vi "Differential Pressure Release Valve Test DAA.vi"(8 "error in (no error)":errorcluster, 10 "Model in":refnum<class "Model.lvclass">, 11 "Test Actuator State in":refnum<class "Test Actuator State.lvclass">) -> (0 "error out":errorcluster, 1 "Pass":bool, 2 "Model out":refnum<class "Model.lvclass">, 3 "Test Actuator State out":refnum<class "Test Actuator State.lvclass">)   [LabVIEW 2016]
uses:
  Model/Model/Model.lvclass
  Typedefs/ActuatorSetPoints.ctl
  <vilib>/platform/TimedLoop/XDataNode/XDataNode.xnode
  <vilib>/Platform/TimedLoop/XDataNode/nitl_modes.ctl
  <vilib>/Platform/TimedLoop/XDataNode/XDNodeRunTimeDep.lvlib
  <vilib>/Platform/TimedLoop/XDataNode/wakeup.ctl
  <vilib>/Platform/TimedLoop/XDataNode/timing_clust.ctl
  Test Actuator State.lvclass
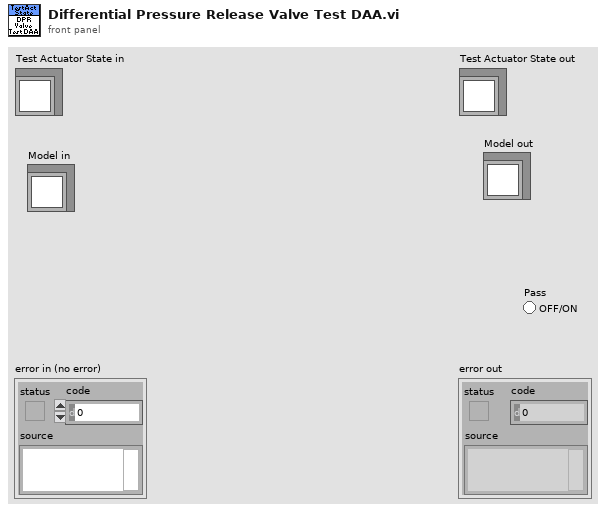
[diagram p1: front panel]
types:
  T1 = typedef "DifferentialPressureReleaseValveTestSettings.ctl" = cluster{"Max Over Force (N)":dbl, "Max Moment (NM)":dbl, "Process Time (s)":dbl, "Sample Time (s)":dbl}
  T2 = typedef "ForcePair.ctl" = cluster{"Axial Force":dbl, "Lateral Force":dbl}
  T3 = typedef "FullForceScanSettings.ctl" = cluster{"Force Tolerance (N)":dbl, "DAA Force Set Points":T2[], "Process Time (s)":dbl, "Sample Time (s)":dbl, "Max Moment (NM)":dbl, "SAA Force Set Points":T2[]}
  T4 = cluster{"Top Left":T2, "Top Right":T2, "Bottom Right":T2, "Bottom Left":T2}
  T5 = typedef "ActuatorSetPoints.ctl" = cluster{"Axial Force":dbl, "Lateral Force":dbl, "FC1 Force":dbl, "FC2 Force":dbl}
  T6 = typedef "XDNodeRunTimeDep.lvlib/timing_clust.ctl" = cluster{"Expected End [f-1]":u64, "Actual End [f-1]":u64, "Finished Late? [f-1]":bool, "Expected End [i-1]":u64, "Actual End [i-1]":u64, "Finished Late? [i-1]":bool, "Expected Start [i]":u64, "Actual Start [i]":u64, "Expected Start [f]":u64, "Actual Start [f]":u64, "Source Name":string, "Structure Name":string, "Period":i64, "Deadline":i64, "Offset":i64, "Start":i64, "Priority":i32, "Timeout":i32, "Mode":T7, "Wakeup Reason":T8, "Error":errorcluster, "Source Type":string, "Secondary Source Type":string, "Global End Time":u64, "Global Start Time":u64, "Frame Duration":u64, "Iteration Duration":u64, "Assigned CPU":i32, "I/O Scan Engine Mode":u32}
  T7 = typedef "XDNodeRunTimeDep.lvlib/nitl_modes.ctl" = enum32{"No Change", "Process missed periods, maintain original phase", "Discard missed periods, maintain original phase", "Process missed periods, ignore original phase", "Discard missed periods, ignore original phase"}
  T8 = typedef "XDNodeRunTimeDep.lvlib/wakeup.ctl" = enum32{"Normal", "Aborted", "Asynchronous wakeup", "Timing source error", "Timed loop error", "Timeout"}
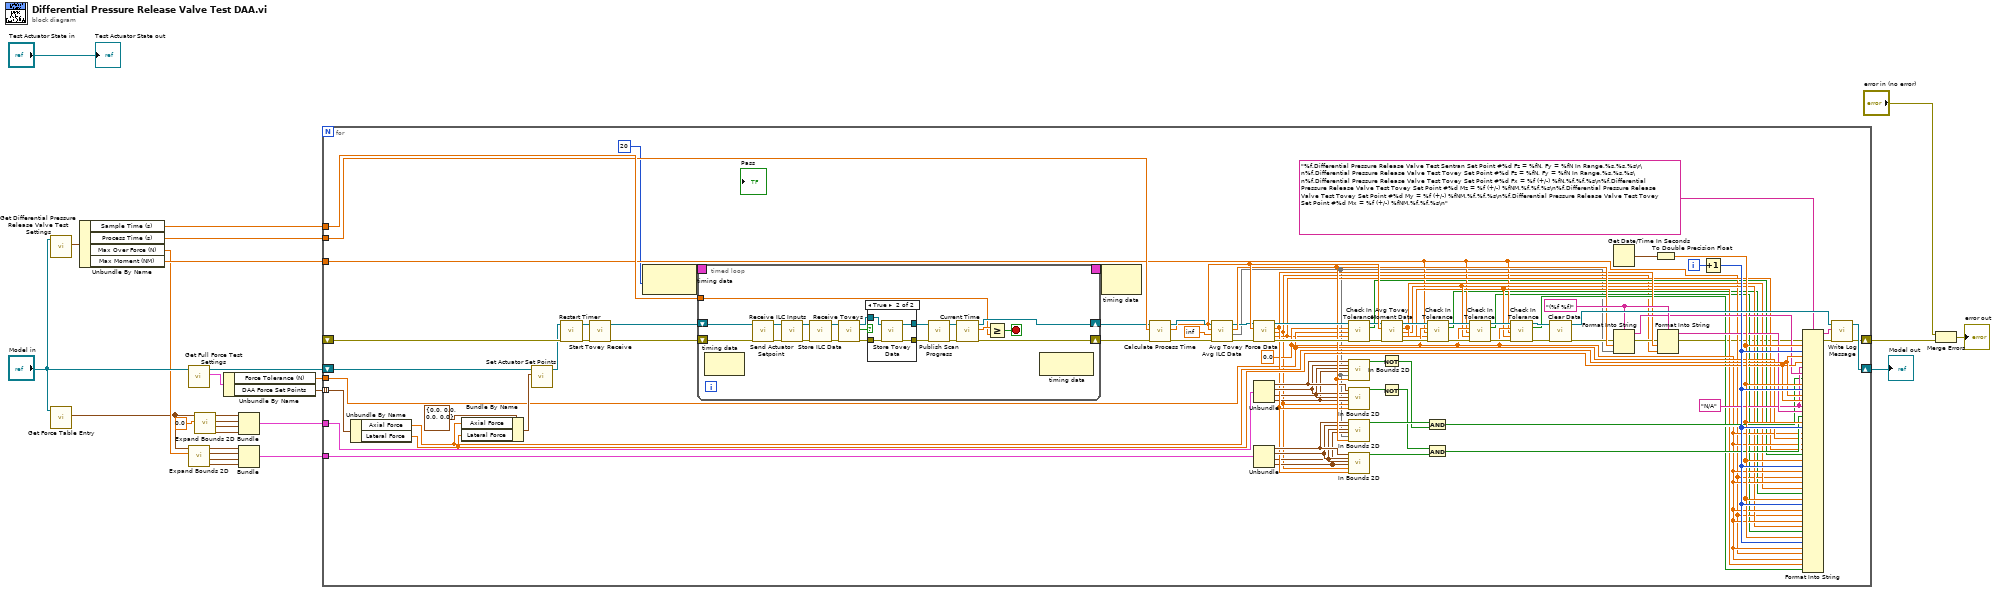
[diagram p0: block diagram]
diagram:
  n1 = call-dynamic "Get Differential Pressure Release Valve Test Settings.vi"("Model in"="Model in") -> ("Differential Pressure Release Valve Test Settings"=w16:T1)  [unwired: 9 in, 1 out]
  n2 = call "Get Force Table Entry.vi"("Model in"="Model in") -> ("Entry"=w8:T2[])  [unwired: 8 in, 2 out]
  n3 = Unbundle By Name(w16) -> ("Sample Time (s)"=w25:dbl, "Process Time (s)"=w24:dbl, "Max Over Force (N)"=w15:dbl, "Max Moment (NM)"=w19:dbl)
  n4 = call "Get Full Force Test Settings.vi"("Model in"="Model in") -> ("Full Force Test Settings"=w18:T3, "Model out"=w26:refnum<class "Model.lvclass">)  [unwired: 9 in]
  n5 = call "Expand Bounds 2D.vi"("Tolerance (N)"=w15, "Entry"=w8) -> ("Bottom Left"=w10:T2, "Bottom Right"=w11:T2, "Top Right"=w12:T2, "Top Left"=w13:T2)  [unwired: 6 in]
  n6 = call "Expand Bounds 2D.vi"("Tolerance (N)"=0.0, "Entry"=w8) -> ("Bottom Left"=w3:T2, "Bottom Right"=w4:T2, "Top Right"=w5:T2, "Top Left"=w6:T2)  [unwired: 6 in]
  n7 = Unbundle By Name(w18) -> ("Force Tolerance (N)"=w1:dbl, "DAA Force Set Points"=w14:T2[])
  n8 = Bundle("Top Left"=w6, "Top Right"=w5, "Bottom Right"=w4, "Bottom Left"=w3) -> (w2:T4)  [unwired: 1 in]
  n9 = Bundle("Top Left"=w13, "Top Right"=w12, "Bottom Right"=w11, "Bottom Left"=w10) -> (w9:T4)  [unwired: 1 in]
  n10 = for {
    tunnel: w14 -> [w99] mode=indexing
    shift-right: [w109] -> w21
    shift-left: w26 -> [w113]
    tunnel: w25 -> [w112]
    tunnel: w24 -> [w95]
    shift-right: [w96] -> w20
    shift-left: _ -> [w111]
    tunnel: w19 -> [w45]
    tunnel: w9 -> [w74]
    tunnel: w2 -> [w73]
    tunnel: w1 -> [w52]
    i -> [w106]
    w63 = "N/A" ("input 5")
    w67 = "(%f %f)" ("format string")
    w50 = 0.0
    n11 = Unbundle By Name(w99) -> ("Axial Force"=w69:dbl, "Lateral Force"=w68:dbl)
    n12 = Bundle By Name(cluster=T5 {"Axial Force"=0.0, "Lateral Force"=0.0, "FC1 Force"=0.0, "FC2 Force"=0.0} ("Actuator Set Points"), "Axial Force"=w69, "Lateral Force"=w68) -> (w100:T5)
    n13 = call "Set Actuator Set Points.vi"("Actuator Set Points"=w100, "Model in"=w113) -> ("Model out"=w101:refnum<class "Model.lvclass">)  [unwired: 9 in]
    n14 = call "Restart Timer.vi"("error in (no error)"=w111, "Model in"=w101) -> ("error out"=w104:errorcluster, "Model out"=w105:refnum<class "Model.lvclass">)  [unwired: 8 in]
    n15 = call "Start Tovey Receive.vi"("error in (no error)"=w104, "Model in"=w105) -> ("error out"=w102:errorcluster, "Model out"=w103:refnum<class "Model.lvclass">)  [unwired: 8 in]
    n16 = node-c288(i64 20 ("Period")) -> (w30:T6)
    n17 = timed-loop {
      shift-right: [w128] -> w94
      shift-left: w103 -> [w134]
      shift-right: [w127] -> w92
      shift-left: w102 -> [w131]
      tunnel: w112 -> [w125]
      timing: w30 -> [_]
      timing-out: [_] -> w29
      stop <- w124 stop-if-true
      n18 = node-c288() -> ()  [unwired: 1 in, 1 out]
      n19 = call "Send Actuator Setpoint.vi"("error in (no error)"=w131, "Model in"=w134) -> ("error out"=w130:errorcluster, "Model out"=w133:refnum<class "Model.lvclass">)  [unwired: 8 in]
      n20 = call "Receive ILC Inputs.vi"("error in (no error)"=w130, "Model in"=w133) -> ("error out"=w129:errorcluster, "Model out"=w132:refnum<class "Model.lvclass">)  [unwired: 8 in]
      n21 = call "Store ILC Data.vi"("error in (no error)"=w129, "Model in"=w132) -> ("error out"=w122:errorcluster, "Model out"=w123:refnum<class "Model.lvclass">)  [unwired: 8 in]
      n22 = call "Receive Toveys.vi"("error in (no error)"=w122, "Model in"=w123) -> ("error out"=w120:errorcluster, "Data Received"=w119:bool, "Model out"=w121:refnum<class "Model.lvclass">)  [unwired: 7 in]
      n23 = case shown="True" w119 {
        tunnel: w121 -> [w138 w142]
        tunnel: w120 -> [w137 w141]
        tunnel: [w137 w140] -> w115
        tunnel: [w138 w139] -> w118
        frame False {
        }
        frame True {
          n24 = call "Store Tovey Data.vi"("error in (no error)"=w141, "Model in"=w142) -> ("error out"=w140:errorcluster, "Model out"=w139:refnum<class "Model.lvclass">)  [unwired: 8 in]
        }
      }
      n25 = call "Publish Scan Progress.vi"("error in (no error)"=w115, "Model in"=w118) -> ("error out"=w116:errorcluster, "Model out"=w117:refnum<class "Model.lvclass">)  [unwired: 8 in]
      n26 = call "Current Time.vi"("error in (no error)"=w116, "Model in"=w117) -> ("error out"=w127:errorcluster, "Time"=w126:dbl, "Model out"=w128:refnum<class "Model.lvclass">)  [unwired: 7 in]
      n27 = Greater Or Equal?(x=w126, y=w125) -> (x >= y?=w124:bool)
      n28 = node-c288() -> ()  [unwired: 1 in, 1 out]
    }
    n29 = node-c288(w29) -> ()  [unwired: 1 out]
    n30 = call "Calculate Process Time.vi"("error in (no error)"=w92, "Seconds"=w95, "Model in"=w94) -> ("error out"=w91:errorcluster, "Time"=w90:dbl, "Model out"=w93:refnum<class "Model.lvclass">)  [unwired: 6 in]
    n31 = call "Avg ILC Data.vi"("error in (no error)"=w91, "Before This Time"=inf, "After This Time"=w90, "Model in"=w93) -> ("error out"=w89:errorcluster, 1:w32, "Force"=w66:dbl, "Model out"=w51:refnum<class "Model.lvclass">)  [unwired: 4 in]
    n32 = call "Avg Tovey Force Data.vi"("Model in"=w51, "After This Time"=w90, "error in (no error)"=w89) -> ("Model out"=w86:refnum<class "Model.lvclass">, "Fz"=w57:dbl, "Fy"=w33:dbl, "Fx"=w49:dbl, "error out"=w85:errorcluster)  [unwired: 8 in]
    n33 = Unbundle(w73) -> ("Top Left"=w59:T2, "Top Right"=w58:T2, "Bottom Right"=w35:T2, "Bottom Left"=w34:T2)
    n34 = Unbundle(w74) -> ("Top Left"=w61:T2, "Top Right"=w60:T2, "Bottom Right"=w37:T2, "Bottom Left"=w36:T2)
    n35 = call "Check In Tolerance.vi"("Model in"=w86, "Expected"=w50, "Tolerance"=w52, "Actual"=w49, "error in (no error)"=w85) -> ("Model out"=w83:refnum<class "Model.lvclass">, "Pass"=w41:bool, "error out"=w84:errorcluster)  [unwired: 8 in]
    n36 = call "In Bounds 2D.vi"("Top Left"=w59, "Top Right"=w58, "Bottom Right"=w35, "Bottom Left"=w34, "Lateral"=w32, "Axial"=w66) -> ("InBounds"=w72:bool)  [unwired: 13 in]
    n37 = call "In Bounds 2D.vi"("Top Left"=w59, "Top Right"=w58, "Bottom Right"=w35, "Bottom Left"=w34, "Lateral"=w33, "Axial"=w57) -> ("InBounds"=w56:bool)  [unwired: 13 in]
    n38 = call "In Bounds 2D.vi"("Top Left"=w61, "Top Right"=w60, "Bottom Right"=w37, "Bottom Left"=w36, "Lateral"=w32, "Axial"=w66) -> ("InBounds"=w71:bool)  [unwired: 13 in]
    n39 = call "In Bounds 2D.vi"("Top Left"=w61, "Top Right"=w60, "Bottom Right"=w37, "Bottom Left"=w36, "Lateral"=w33, "Axial"=w57) -> ("InBounds"=w54:bool)  [unwired: 13 in]
    n40 = Not(x=w72) -> (.not. x?=w70:bool)
    n41 = Not(x=w56) -> (.not. x?=w55:bool)
    n42 = call "Avg Tovey Moment Data.vi"("Model in"=w83, "After This Time"=w90, "error in (no error)"=w84) -> ("Model out"=w82:refnum<class "Model.lvclass">, "Mz"=w48:dbl, "My"=w47:dbl, "Mx"=w46:dbl, "error out"=w81:errorcluster)  [unwired: 8 in]
    n43 = And(x=w71, y=w70) -> (x .and. y?=w62:bool)
    n44 = And(x=w55, y=w54) -> (x .and. y?=w53:bool)
    n45 = call "Check In Tolerance.vi"("Model in"=w82, "Expected"=w50, "Tolerance"=w45, "Actual"=w48, "error in (no error)"=w81) -> ("Model out"=w80:refnum<class "Model.lvclass">, "Pass"=w42:bool, "error out"=w77:errorcluster)  [unwired: 8 in]
    n46 = call "Check In Tolerance.vi"("Model in"=w80, "Expected"=w50, "Tolerance"=w45, "Actual"=w47, "error in (no error)"=w77) -> ("Model out"=w79:refnum<class "Model.lvclass">, "Pass"=w43:bool, "error out"=w76:errorcluster)  [unwired: 8 in]
    n47 = call "Check In Tolerance.vi"("Model in"=w79, "Expected"=w50, "Tolerance"=w45, "Actual"=w46, "error in (no error)"=w76) -> ("Model out"=w78:refnum<class "Model.lvclass">, "Pass"=w44:bool, "error out"=w75:errorcluster)  [unwired: 8 in]
    n48 = call "Clear Data.vi"("error in (no error)"=w75, "Model in"=w78) -> ("error out"=w40:errorcluster, "Model out"=w110:refnum<class "Model.lvclass">)  [unwired: 8 in]
    n49 = Get Date/Time In Seconds() -> (seconds since 1Jan1904=w107:timestamp)
    n50 = Format Into String(format string=w67, error in=w40, w66, w32) -> (resulting string=w65:string, error out=w39:errorcluster)  [unwired: 1 in]
    n51 = To Double Precision Float(number=w107) -> (double precision float=w87:dbl)
    n52 = Format Into String(format string=w67, error in=w39, w57, w33) -> (resulting string=w64:string, error out=w38:errorcluster)  [unwired: 1 in]
    n53 = Increment(x=w106) -> (x+1=w88:i32)
    n54 = Format Into String(format string="%f,Differential Pressure Release Valve Test Sentran Set Point #%d Fz = %fN, Fy = %fN In Range,%s,%s,%s\r\n%f,Differential Pressure Release Valve Test Tovey Set Point #%d Fz = %fN, Fy = %fN In Range,%s,%s,%s\n%f,Differential Pressure Release Valve Test Tovey Set Point #%d Fx = %f (+/-) %fN,%f,%f,%s\n%f,Differential Pressure Release Valve Test Tovey Set Point #%d Mz = %f (+/-) %fNM,%f,%f,%s\n%f,Differential Pressure Release Valve Test Tovey Set Point #%d My = %f (+/-) %fNM,%f,%f,%s\n%f,Differential Pressure Release Valve Test Tovey Set Point #%d Mx = %f (+/-) %fNM,%f,%f,%s\n", error in=w38, w87, w88, w69, w68, w63, w65, w62, w87, w88, w69, w68, w63, w64, w53, w87, w88, w50, w52, w50, w49, w41, w87, w88, w50, w45, w50, w48, w42, w87, w88, w50, w45, w50, w47, w43, w87, w88, w50, w45, w50, w46, w44) -> (resulting string=w98:string, error out=w97:errorcluster)  [unwired: 1 in]
    n55 = call "Write Log Message.vi"("error in (no error)"=w97, "Message"=w98, "Model in"=w110) -> ("error out"=w96:errorcluster, "Model out"=w109:refnum<class "Model.lvclass">)  [unwired: 7 in]
  }
  "Model out" <- w21
  n56 = Merge Errors("error in (no error)", w20) -> (→"error out":errorcluster)
  "Test Actuator State out" <- "Test Actuator State in"
